vi "FPGA Inverse Time Delay (Dependent Reset).vi"(0 "pick-up signal? (F)":bool, 1 "number of channels":T2=1 items=["1"=1, "2"=2, "3"=3, "4"=4, "5"=5, "6"=6, "7"=7, "8"=8, "9"=9, "10"=10, "11"=11, "12"=12, "13"=13, "14"=14, "15"=15, "16"=16], 2 "memory info of curve":T1={"reference"="", "size"=240}, 5 "G":fxp<+/-,48,24>, 7 "Gs":fxp<+/-,48,24>, 9 "input valid? (T)":bool=TRUE, 12 "ready for output? (T)":bool=TRUE, 13 "instantaneous reset after tripping? (F)":bool) -> (4 "trip signal?":bool, 10 "output valid?":bool, 14 "ready for input?":bool, 15 "error":i32)   [LabVIEW 2013, in "NI_EP_Protection_FPGA.lvlib"]
doc: "Delays for the time interval that you specify in the Inverse Time Curves VI before the trip signal asserts. The Inverse Time Curves VI generates inverse time curves for this VI to use. You can compensate for the processing delay of the input energizing quantity under a specific G/Gs in the Inverse Time Curves VI to achieve higher operate time accuracy."
uses:
  <vilib>/addons/Electrical Power/Protection/NI_EP_Protection_FPGA.lvlib
  <vilib>/addons/Electrical Power/PQ/Resampling/FPGA/subVIs/fpga_NofCH.ctl
  <vilib>/addons/Electrical Power/Protection/Inverse Time Delay/subVIs/ep_Curve Memory.ctl
  <vilib>/rvi/FXPMathLib/basic elements/FxpDiscreteDelay/XNode/nifxpmath_DiscreteDelay.xnode
  <vilib>/addons/Electrical Power/PQ/Resampling/NI_EP_Resample_FPGA.lvlib
  <vilib>/addons/Electrical Power/Protection/NI_EP_Protection.lvlib
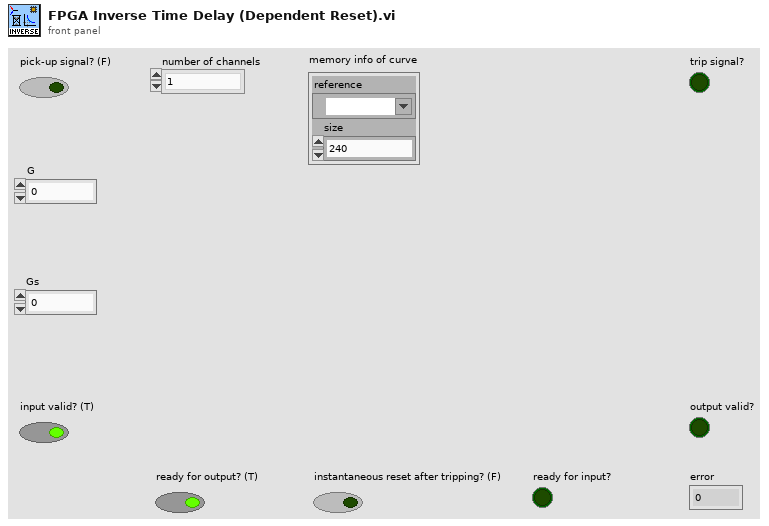
[diagram p1: front panel]
types:
  T1 = typedef "NI_EP_Protection.lvlib/ep_Curve Memory.ctl" = cluster{"reference":refnum<k21>, "size":u16}
  T2 = typedef "NI_EP_Resample_FPGA.lvlib/fpga_NofCH.ctl" = u8
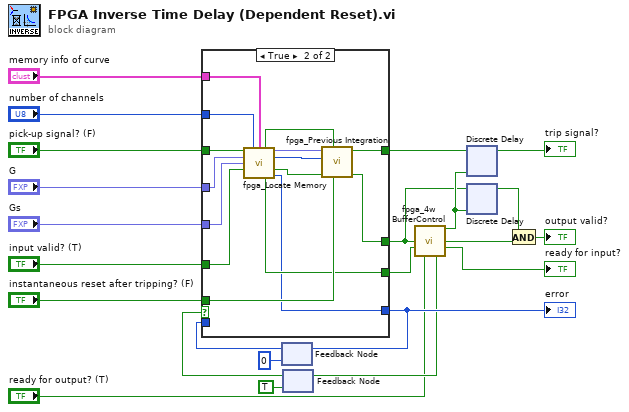
[diagram p0: block diagram]
diagram:
  n1 = feedback #1(0 ("code")) -> (w8:i32)
  n2 = feedback #2(TRUE ("logic enable")) -> (w11:bool)
  n3 = case shown="True" w11 {
    tunnel: "number of channels" -> [_ w36]
    tunnel: "instantaneous reset after tripping? (F)" -> [_ w39]
    tunnel: "memory info of curve" -> [_ w35]
    tunnel: [_ w38] -> w13
    tunnel: "G" -> [_ w33]
    tunnel: "Gs" -> [_ w32]
    tunnel: "input valid? (T)" -> [_ w31]
    tunnel: "pick-up signal? (F)" -> [_ w34]
    tunnel: [w24 w25] -> w9
    tunnel: [_ w37] -> w14
    tunnel: w8 -> [w24 _]
    tunnel: [_ w26] -> w6
    frame False {
    }
    frame True {
      n4 = call <vilib>:"fpga_Locate Memory.vi"("pick-up signal? (F)"=w34, "number of channels"=w36, "memory info of curve"=w35, "G"=w33, "Gs"=w32, "input valid? (T)"=w31) -> ("integrate?"=w27:bool, "dt/T"=w30:fxp<+/-,32,1>, "channel index"=w29:u8, "output valid"=w28:bool, "ready for input"=w26:bool, "error"=w25:i32)  [unwired: 3 in, 1 out]
      n5 = call <vilib>:"fpga_Previous Integration.vi"("instantaneous reset after tripping? (F)"=w39, "integrate?"=w27, "input valid"=w28, "channel index"=w29, "dt/T"=w30) -> ("output valid"=w38:bool, "trip?"=w37:bool)  [unwired: 4 in, 1 out]
    }
  }
  "error" <- w9
  n6 = feedback-in #1(w9) -> ()
  n7 = call <vilib>:"fpga_4w BufferControl.vi"("DR"=w13, "RFI"=w6, "RFO"="ready for output? (T)") -> ("buff enable"=w16:bool, "output valid"=w15:bool, "ready for input"=→"ready for input?":bool, "logic enable"=w5:bool)  [unwired: 9 in]
  n8 = feedback-in #2(w5) -> ()
  n9 = xnode ("Discrete Delay")("D"=w14, "enable"=w16) -> ("Q"=→"trip signal?":bool)
  n10 = xnode ("Discrete Delay")("D"=w13, "enable"=w16) -> ("Q"=w12:bool)
  n11 = And(x=w12, y=w15) -> (x .and. y?=→"output valid?":bool)
